vi "Scanstep.per.monoStep.vi"(10 "Mono in":T2, 11 "DyeLaser":T1={"Scan.Start (cm-1)"=15000.0, "Scan.Stop (cm-1)"=15050.0, "Scan.step (cm-1)"=0.2, "VISA resource name"="", "Laser"=enum."Syrah", "NSteps"=251, "CurrentStep"=75, "Current.cm-1"=15015.0} {"Current.cm-1" format="%.2f"}) -> (2 "Mono out":T2, 3 "DyeLaser out":T1={"Scan.Start (cm-1)"=15000.0, "Scan.Stop (cm-1)"=15050.0, "Scan.step (cm-1)"=0.2, "VISA resource name"="", "Laser"=enum."Syrah", "NSteps"=251, "CurrentStep"=75, "Current.cm-1"=15015.0} {"Current.cm-1" format="%.2f"})   [LabVIEW 2022 SP3]
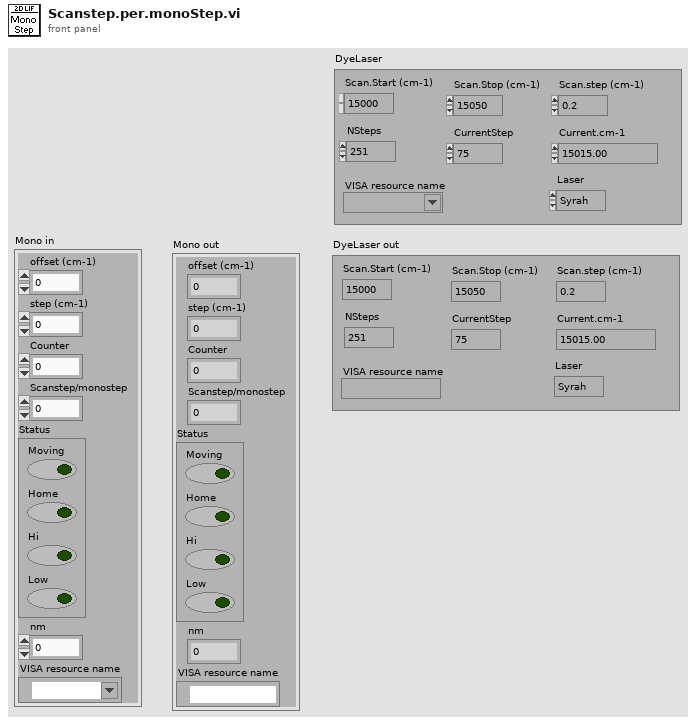
[diagram p1: front panel]
types:
  T1 = cluster{"Scan.Start (cm-1)":dbl, "Scan.Stop (cm-1)":dbl, "Scan.step (cm-1)":dbl, "VISA resource name":refnum<visa-resource-name>, "Laser":enum16{"Syrah", "Hyperdye"}, "NSteps":i32, "CurrentStep":i32, "Current.cm-1":dbl}
  T2 = cluster{"offset (cm-1)":dbl, "step (cm-1)":dbl, "Counter":dbl, "Scanstep/monostep":i32, "Status":cluster{"Moving":bool, "Home":bool, "Hi":bool, "Low":bool}, "nm":dbl, "VISA resource name":refnum<visa-resource-name>}
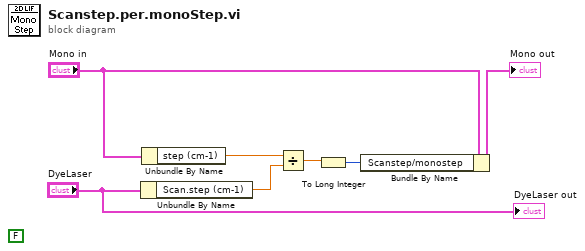
[diagram p0: block diagram]
diagram:
  (unwired) FALSE ("Status.Moving")
  n1 = Unbundle By Name("DyeLaser") -> ("Scan.step (cm-1)"=w4:dbl)
  n2 = Unbundle By Name("Mono in") -> ("step (cm-1)"=w6:dbl)
  n3 = Divide(x=w6, y=w4) -> (x/y=w1:dbl)
  n4 = To Long Integer(number=w1) -> (32bit integer=w2:i32)
  n5 = Bundle By Name(cluster="Mono in", "Scanstep/monostep"=w2) -> (→"Mono out":T2)
  "DyeLaser out" <- "DyeLaser"
